vi "get desired keys.vi"(8 "error in":errorcluster, 11 "CentralErrorHandlerDev configuration in":refnum<class "CentralErrorHandler configuration.lvclass">) -> (0 "error out":errorcluster, 2 "desired keys":string[](array[string]), 3 "CentralErrorHandlerDev configuration out":refnum<class "CentralErrorHandler configuration.lvclass">)   [LabVIEW 2017, in "CentralErrorHandler configuration.lvclass"]
uses:
  CentralErrorHandler configuration.lvclass
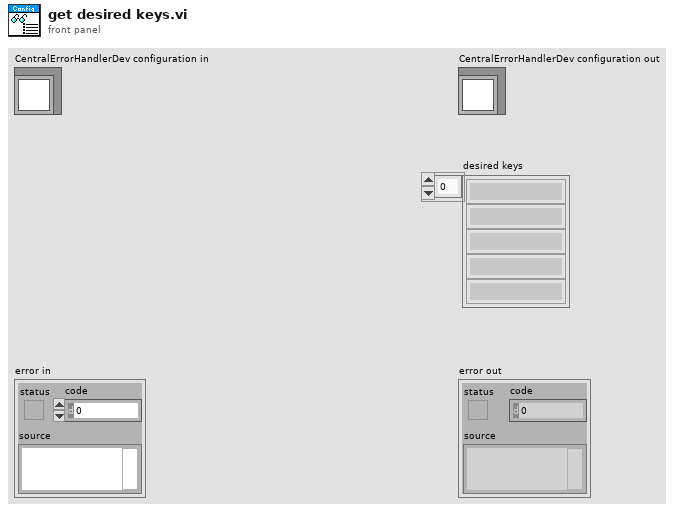
[diagram p1: front panel]
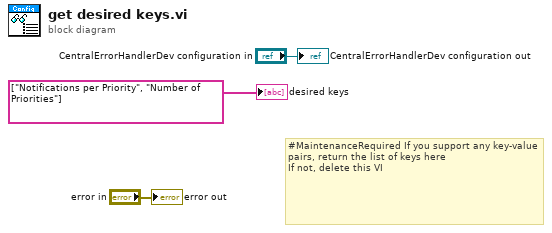
[diagram p0: block diagram]
diagram:
  # "#MaintenanceRequired If you support any key-value pairs, return the list of keys here\nIf not, delete this VI"
  "error out" <- "error in"
  "CentralErrorHandlerDev configuration out" <- "CentralErrorHandlerDev configuration in"
  "desired keys" <- string[] ["Notifications per Priority", "Number of Priorities"] ("desired keys")
